vi "APDM Open All APs.vi"(2 "error in (no error)":errorcluster, 3 "APDM Context":T1={"APDM Context ID"=0, "Gyro Mode"="", "Log Data"=FALSE, "Log File"=refnum, "Gyro Record Log"=refnum, "Gyro CMD Log"=refnum, "L Opal SN"=0, "R Opal SN"=0, "Access Point ID"=0, "Left Gyro Sim Data"=path "C:/Users/jfalesi/Desktop/CP FES Walking Code/Original/Ahad Vi/CP Code/Offline data/TD_7_Raw_R.txt", "Right Gyro Sim Data"=path "C:/Users/jfalesi/Desktop/CP FES Walking Code/Original/Ahad Vi/CP Code/Offline data/TD_7_Raw_R.txt", "Sampling Rate"=0.0, "Gyro Sim Time Array"=[], "Missed Gyro Count"=0.0}) -> (0 "error out":errorcluster, 1 "APDM Context":T1={"APDM Context ID"=0, "Gyro Mode"="", "Log Data"=FALSE, "Log File"=refnum, "Gyro Record Log"=refnum, "Gyro CMD Log"=refnum, "L Opal SN"=0, "R Opal SN"=0, "Access Point ID"=0, "Left Gyro Sim Data"=path "C:/Users/jfalesi/Desktop/CP FES Walking Code/Original/Ahad Vi/CP Code/Offline data/TD_7_Raw_R.txt", "Right Gyro Sim Data"=path "C:/Users/jfalesi/Desktop/CP FES Walking Code/Original/Ahad Vi/CP Code/Offline data/TD_7_Raw_R.txt", "Sampling Rate"=0.0, "Gyro Sim Time Array"=[], "Missed Gyro Count"=0.0})   [LabVIEW 2019]
uses:
  Controls/APDM Context Cluster.ctl
  Program Files/National Instruments/LabVIEW 2019/user.lib/apdm/apdm.lvlib
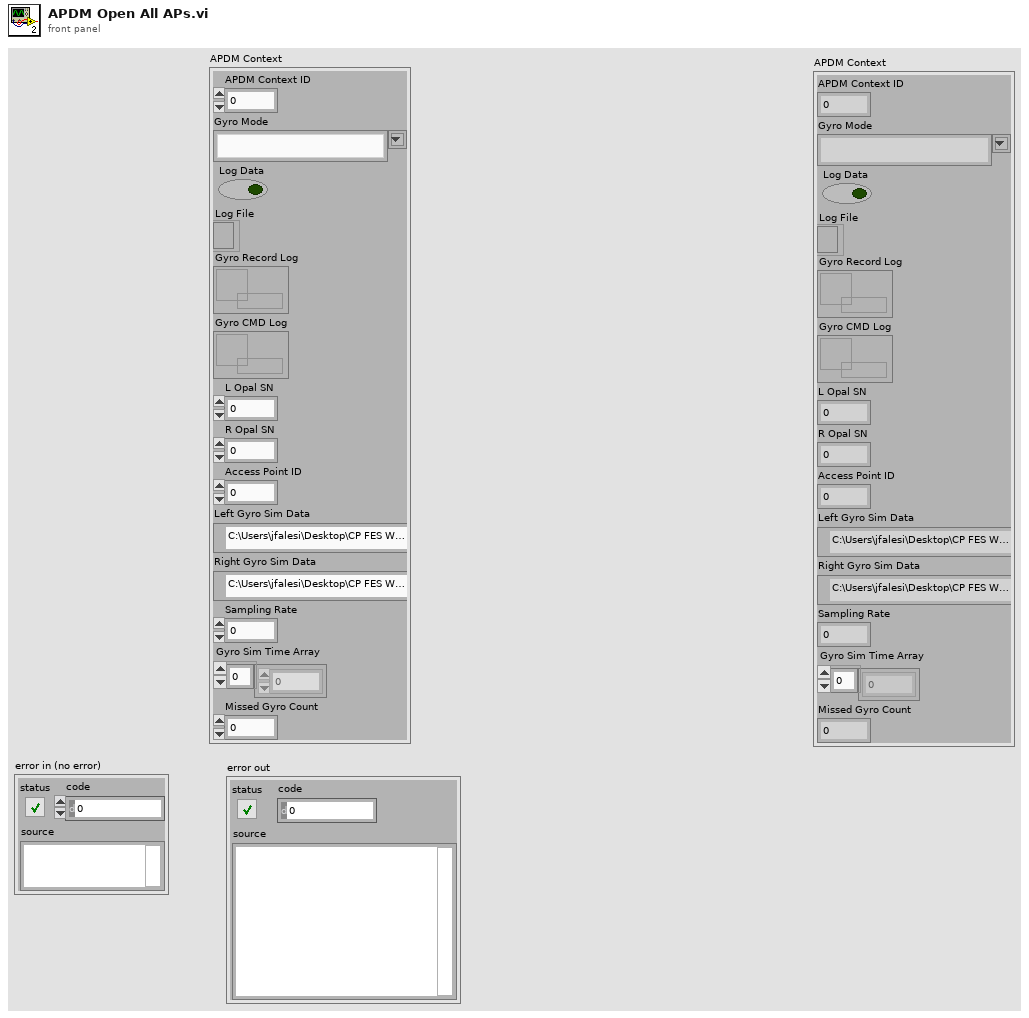
[diagram p1: front panel]
types:
  T1 = typedef "APDM Context Cluster.ctl" = cluster{"APDM Context ID":u32, "Gyro Mode":string, "Log Data":bool, "Log File":refnum<file>, "Gyro Record Log":refnum<queue>, "Gyro CMD Log":refnum<queue>, "L Opal SN":u32, "R Opal SN":u32, "Access Point ID":u32, "Left Gyro Sim Data":path, "Right Gyro Sim Data":path, "Sampling Rate":dbl, "Gyro Sim Time Array":dbl[], "Missed Gyro Count":dbl}
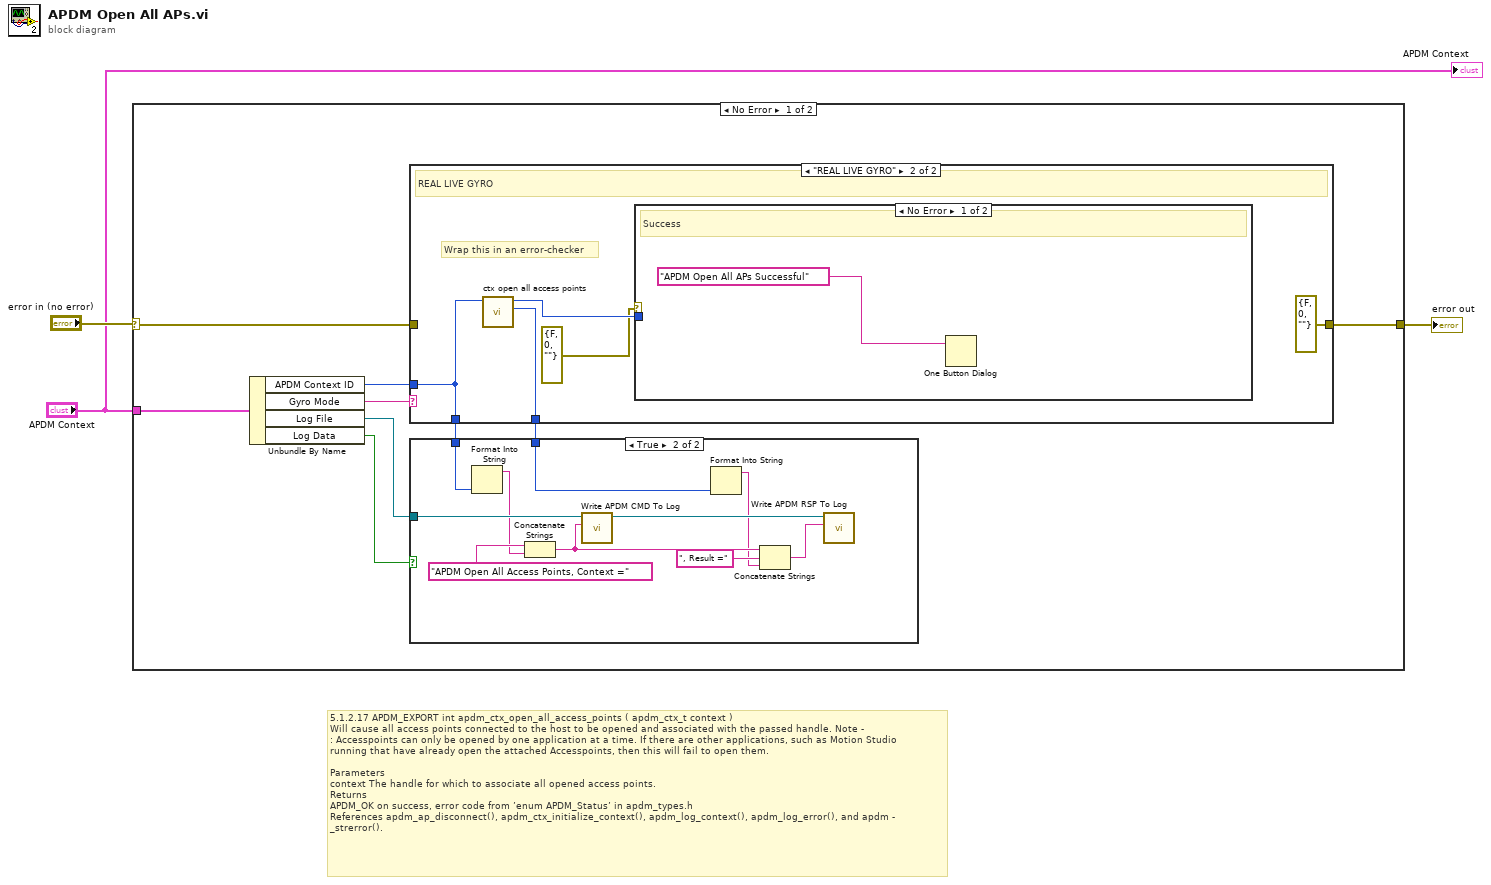
[diagram p0: block diagram]
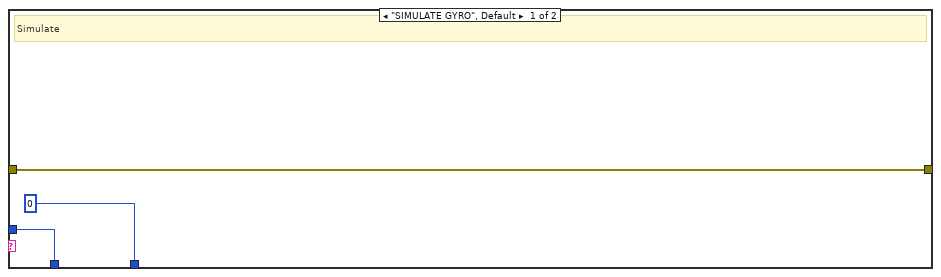
[diagram p3: hidden frame]
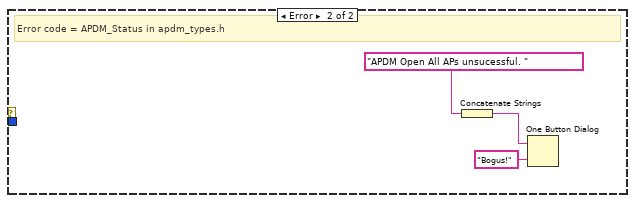
[diagram p4: hidden frame]
diagram:
  # "5.1.2.17 APDM_EXPORT int apdm_ctx_open_all_access_points ( apdm_ctx_t context )\nWill cause all access points connected to the host to be opened and associated with the passed handle. Note -\n: Accesspoints can only be opened by one application at a time. If there are other applications, such as Motion Studio\nrunning that have already open the attached Accesspoints, then this will fail to open them.\n\nParameters\ncontext The handle for which to associate all opened access points.\nReturns\nAPDM_OK on success, error code from ’enum APDM_Status’ in apdm_types.h\nReferences apdm_ap_disconnect(), apdm_ctx_initialize_context(), apdm_log_context(), apdm_log_error(), and apdm -\n_strerror()."
  n1 = case shown="No Error" "error in (no error)" {
    selector: "error in (no error)" -> [w5 w35]
    tunnel: [w12 w35] -> w3
    tunnel: "APDM Context" -> [w4 _]
    frame No Error {
      n2 = Unbundle By Name(w4) -> ("APDM Context ID"=w10:u32, "Gyro Mode"=w9:string, "Log File"=w7:refnum<file>, "Log Data"=w8:bool)
      n3 = case shown="\"REAL LIVE GYRO\"" w9 {
        tunnel: w10 -> [w23 w30]
        tunnel: [w25 errorcluster {"status"=FALSE, "code"=0, "source"=""} ("error IO")] -> w12
        tunnel: w5 -> [w25 _]
        tunnel: [0 w29] -> w11
        tunnel: [w23 w30] -> w6
        frame "SIMULATE GYRO", Default {
          # "Simulate"
        }
        frame "REAL LIVE GYRO" {
          # "Wrap this in an error-checker"
          # "REAL LIVE GYRO"
          n4 = call "ctx open all access points.vi"("context"=w30) -> ("function return"=w29:i32, "context out"=w28:u32)  [unwired: 9 in]
          n5 = case shown="No Error" errorcluster {"status"=FALSE, "code"=0, "source"=""} ("error IO") {
            tunnel: w28 -> [_ _]
            frame No Error {
              # "Success"
              n6 = One Button Dialog(message="APDM Open All APs Successful") -> ()  [unwired: 1 in, 1 out]
            }
            frame Error {
              # "Error code = APDM_Status in apdm_types.h"
              n7 = Concatenate Strings("APDM Open All APs unsucessful. " ("message")) -> (w33:string)
              n8 = One Button Dialog(message=w33, button name ("OK")="Bogus!") -> ()  [unwired: 1 out]
            }
          }
        }
      }
      n9 = case shown="True" w8 {
        tunnel: w11 -> [_ w21]
        tunnel: w7 -> [_ w20]
        tunnel: w6 -> [_ w18]
        frame False {
        }
        frame True {
          n10 = Format Into String(w18) -> (resulting string=w17:string)  [unwired: 3 in, 1 out]
          n11 = Concatenate Strings("APDM Open All Access Points, Context =" ("Log Item"), w17) -> (w16:string)
          n12 = call "Write APDM CMD To Log.vi"("Log Item"=w16, "Byte Stream File in"=w20) -> ("Byte Stream File out"=w22:refnum<file>)  [unwired: 8 in, 1 out]
          n13 = Format Into String(w21) -> (resulting string=w14:string)  [unwired: 3 in, 1 out]
          n14 = Concatenate Strings(w16, ", Result =" ("Log Item"), w14) -> (w13:string)
          n15 = call "Write APDM RSP To Log.vi"("Log Item"=w13, "Byte Stream File in"=w22) -> ()  [unwired: 9 in, 1 out]
        }
      }
    }
    frame Error {
    }
  }
  "error out" <- w3
  "APDM Context" <- "APDM Context"
